vi "BMP180 Pull Raw Measurement.vi"(6 "Sensor Type":enum16{"Temp", "Pressure"}(ring), 7 "I2C Channel":u8, 8 "error in (no error)":errorcluster, 9 "BMP180 Config":T7 {"Cal Coefs"."MD"."Val:" format="%04x"; "Cal Coefs"."MD"."Addr:" format="%02x"; "Cal Coefs"."MC"."Val:" format="%04x"; "Cal Coefs"."MC"."Addr:" format="%02x"; "Cal Coefs"."MB"."Val:" format="%04x"; "Cal Coefs"."MB"."Addr:" format="%02x"; "Cal Coefs"."B2"."Val:" format="%04x"; "Cal Coefs"."B2"."Addr:" format="%02x"; "Cal Coefs"."B1"."Val:" format="%04x"; "Cal Coefs"."B1"."Addr:" format="%02x"; "Cal Coefs"."AC6"."Val:" format="%04x"; "Cal Coefs"."AC6"."Addr:" format="%02x"; "Cal Coefs"."AC5"."Val:" format="%04x"; "Cal Coefs"."AC5"."Addr:" format="%02x"; "Cal Coefs"."AC4"."Val:" format="%04x"; "Cal Coefs"."AC4"."Addr:" format="%02x"; "Cal Coefs"."AC3"."Val:" format="%04x"; "Cal Coefs"."AC3"."Addr:" format="%02x"; "Cal Coefs"."AC2"."Val:" format="%04x"; "Cal Coefs"."AC2"."Addr:" format="%02x"; "Cal Coefs"."AC1"."Val:" format="%04x"; "Cal Coefs"."AC1"."Addr:" format="%02x"}, 10 "I2C Slave Address":u8 format="%.0x", 11 "LINX Resource in":T1) -> (0 "error out":errorcluster, 2 "Raw Reading":i32, 3 "LINX Resource":T1)   [LabVIEW 2014]
uses:
  BMP180 Config Options.ctl
  <vilib>/MakerHub/LINX/Private/Type Defs/LINX Ref.ctl
  <vilib>/MakerHub/LINX/Private/Type Defs/Platform.ctl
  <vilib>/MakerHub/LINX/Private/Type Defs/Interface.ctl
  <vilib>/MakerHub/LINX/Private/Device/Type Defs/LINX Device Config.ctl
  <vilib>/MakerHub/LINX/Private/Device/Type Defs/TCP Config.ctl
  <vilib>/MakerHub/LINX/Private/Device/Type Defs/Channels.ctl
  <vilib>/MakerHub/LINX/Private/Local IO/LinxI2cWrite.vi
  <vilib>/MakerHub/LINX/Public/Utilities/Check Channel.vi
  <vilib>/myRIO/Instrument Drivers/Onboard IO/I2C/vis/Write.vi
  <vilib>/MakerHub/LINX/Private/Utilties/Generate Error.vi
  <vilib>/MakerHub/LINX/Private/Utilties/Channel FGVs/I2C Channels.vi
  <vilib>/Utility/error.llb/Error Cluster From Error Code.vi
  <vilib>/myRIO/Common/Instrument Driver Framework/myRIO v1.0/I2C/vis/myRIO v1.0 Write I2C.vi
  <vilib>/MakerHub/LINX/LMH-LINX.lvlib
  <vilib>/MakerHub/LINX/Private/Device/Device.lvlib
panel:
  out "Data":u8[](array[numeric]) format="%.0x"
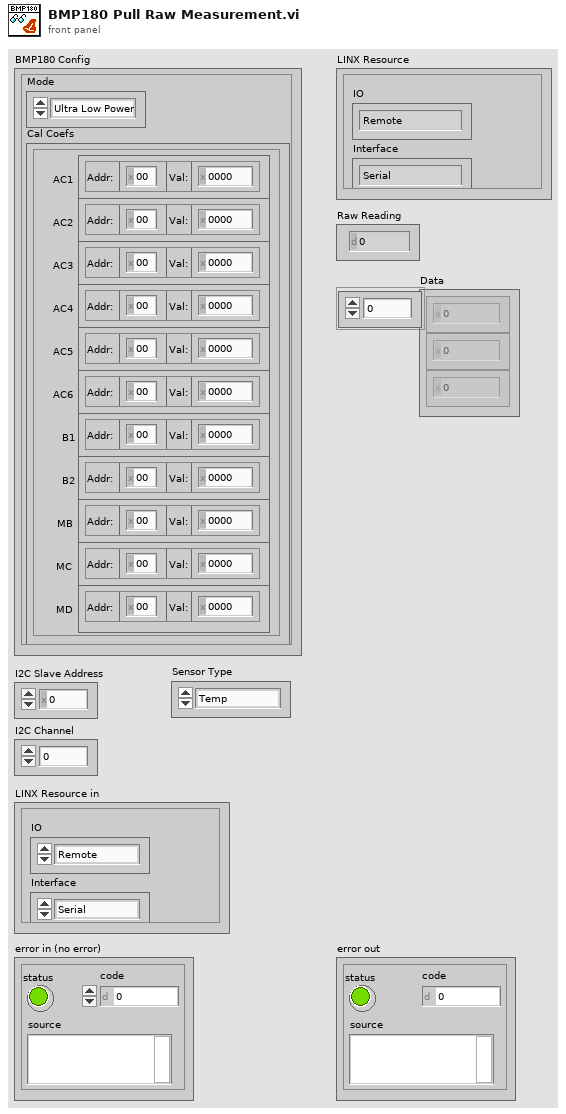
[diagram p1: front panel]
types:
  T1 = typedef "LMH-LINX.lvlib/LINX Ref.ctl" = cluster{"IO":T2, "Interface":T3, "LINX Device Config":T4}
  T2 = typedef "LMH-LINX.lvlib/Platform.ctl" = enum16{"Remote", "Local"}
  T3 = typedef "LMH-LINX.lvlib/Interface.ctl" = enum16{"Serial", "TCP"}
  T4 = typedef "LMH-LINX.lvlib/Device.lvlib/LINX Device Config.ctl" = cluster{"Interface":T3, "COM Port":refnum<visa-resource-name>, "TCP Configuration":T5, "Device Family":u8, "Device ID":u8, "Device Name":string, "TCP Ref":refnum<k5>, "Channels":T6}
  T5 = typedef "LMH-LINX.lvlib/Device.lvlib/TCP Config.ctl" = cluster{"IP Address":string, "Port":u16}
  T6 = typedef "LMH-LINX.lvlib/Channels.ctl" = cluster{"DI":u8[], "DO":u8[], "AI":u8[], "AO":u8[], "PWM":u8[], "QE":u8[], "UART":u8[], "I2C 2":u8[], "SPI":u8[], "CAN":u8[], "Servo":u8[], "AI Ref (V)":dbl, "AI Resolution (Bits)":u8, "AO Ref (V)":dbl, "AO Resolution (Bits)":u8}
  T7 = typedef "BMP180 Config Options.ctl" = cluster{"Mode":enum8{"Ultra Low Power", "Standard", "High Resolution", "Ultra High Resolution"}, "Cal Coefs":cluster{"AC1":cluster{"Addr:":u8, "Val:":u16}, "AC2":cluster{"Addr:":u8, "Val:":u16}, "AC3":cluster{"Addr:":u8, "Val:":u16}, "AC4":cluster{"Addr:":u8, "Val:":u16}, "AC5":cluster{"Addr:":u8, "Val:":u16}, "AC6":cluster{"Addr:":u8, "Val:":u16}, "B1":cluster{"Addr:":u8, "Val:":u16}, "B2":cluster{"Addr:":u8, "Val:":u16}, "MB":cluster{"Addr:":u8, "Val:":u16}, "MC":cluster{"Addr:":u8, "Val:":u16}, "MD":cluster{"Addr:":u8, "Val:":u16}}}
  T8 = enum8{"Ultra Low Power", "Standard", "High Resolution", "Ultra High Resolution"}
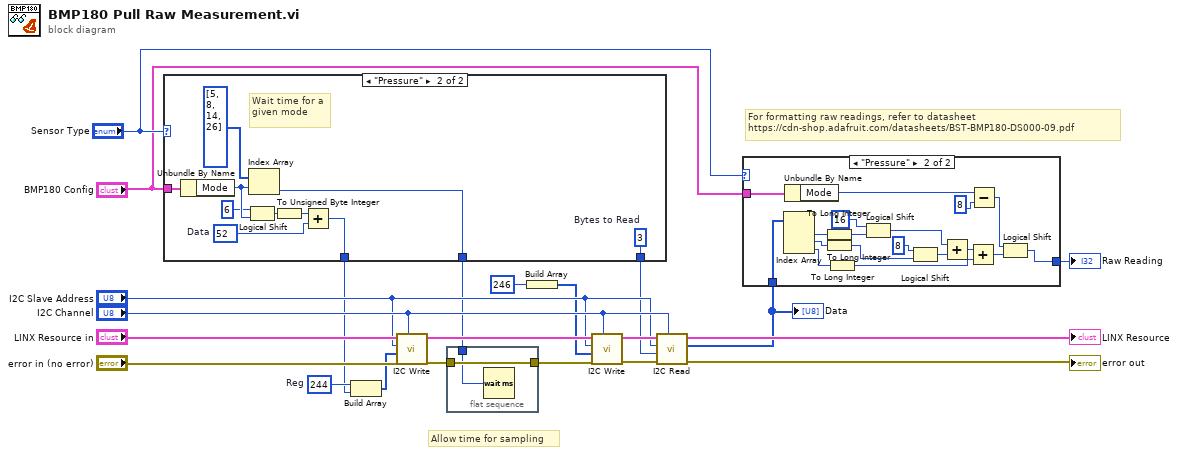
[diagram p0: block diagram]
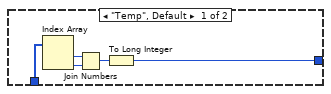
[diagram p2: hidden frame]
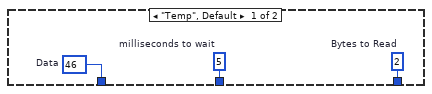
[diagram p3: hidden frame]
diagram:
  w10 = u8 244  # Reg
  # "For formatting raw readings, refer to datasheet\nhttps://cdn-shop.adafruit.com/datasheets/BST-BMP180-DS000-09.pdf"
  # "Allow time for sampling"
  n1 = case shown="\"Pressure\"" "Sensor Type" {
    tunnel: [w25 w33] -> w11
    tunnel: "BMP180 Config" -> [_ w35]
    tunnel: [w24 w27] -> w8
    tunnel: [w23 w26] -> w7
    frame "Temp", Default {
      w23 = u8 2  # Bytes to Read
      w24 = u8 46  # Data
      w25 = u32 5  # milliseconds to wait
    }
    frame "Pressure" {
      w26 = u8 3  # Bytes to Read
      w29 = u8 52  # Data
      # "Wait time for a given mode"
      n2 = Unbundle By Name(w35) -> ("Mode"=w32:T8)
      n3 = Logical Shift(y=i16 6, x=w32) -> (x << y=w30:u32)
      n4 = Index Array(array=u32[] [5, 8, 14, 26], index=w32) -> (element=w33:u32)
      n5 = To Unsigned Byte Integer(number=w30) -> (unsigned 8bit integer=w28:u8)
      n6 = Add(x=w28, y=w29) -> (x+y=w27:u8)
    }
  }
  n7 = Build Array(w10, w8) -> (w9:u8[])
  n8 = call <vilib>:"I2C Write.vi"("I2C Channel"="I2C Channel", "Error In"="error in (no error)", "Data"=w9, "I2C Slave Address (0)"="I2C Slave Address", "LINX Resource"="LINX Resource in") -> ("Error Out"=w18:errorcluster, "LINX Resource"=w19:T1)  [unwired: 5 in]
  n9 = flat-sequence {
    tunnel: [w37] -> w20
    tunnel: w18 -> [w37]
    tunnel: w11 -> [w36]
    frame #0 {
      n10 = Wait (ms)(milliseconds to wait=w36) -> ()  [unwired: 1 out]
    }
  }
  n11 = Build Array(u8 246 ("I2C Slave Address 2")) -> (w2:u8[])
  n12 = call <vilib>:"I2C Write.vi"("I2C Channel"="I2C Channel", "Error In"=w20, "Data"=w2, "I2C Slave Address (0)"="I2C Slave Address", "LINX Resource"=w19) -> ("Error Out"=w21:errorcluster, "LINX Resource"=w22:T1)  [unwired: 5 in]
  n13 = call <vilib>:"I2C Read.vi"("I2C Channel"="I2C Channel", "Error In"=w21, "Bytes To Read"=w7, "I2C Slave Address (0)"="I2C Slave Address", "LINX Resource"=w22) -> ("Error Out"=→"error out":errorcluster, "Data"=w5:u8[], "LINX Resource"=→"LINX Resource":T1)  [unwired: 4 in]
  "Data" <- w5
  n14 = case shown="\"Pressure\"" "Sensor Type" {
    tunnel: w5 -> [w39 w60]
    tunnel: "BMP180 Config" -> [_ w59]
    tunnel: [w38 w43] -> w1
    frame "Temp", Default {
      n15 = Index Array(array=w39) -> (element #1=w42:u8, element #2=w41:u8)  [unwired: 2 in]
      n16 = Join Numbers(hi=w42, lo=w41) -> ((hi.lo)=w40:u16)
      n17 = To Long Integer(number=w40) -> (32bit integer=w38:i32)
    }
    frame "Pressure" {
      n18 = Index Array(array=w60) -> (element #1=w58:u8, element #2=w52:u8, element #3=w50:u8)  [unwired: 3 in]
      n19 = Unbundle By Name(w59) -> ("Mode"=w46:T8)
      n20 = To Long Integer(number=w58) -> (32bit integer=w57:i32)
      n21 = To Long Integer(number=w52) -> (32bit integer=w51:i32)
      n22 = To Long Integer(number=w50) -> (32bit integer=w49:i32)
      n23 = Logical Shift(y=i16 16, x=w57) -> (x << y=w54:i32)
      n24 = Logical Shift(y=i16 8, x=w51) -> (x << y=w55:i32)
      n25 = Add(x=w54, y=w55) -> (x+y=w48:i32)
      n26 = Add(x=w48, y=w49) -> (x+y=w47:i32)
      n27 = Subtract(x=w46, y=i16 8) -> (x-y=w44:i16)
      n28 = Logical Shift(y=w44, x=w47) -> (x << y=w43:i32)
    }
  }
  "Raw Reading" <- w1
